vi "Scpi_srend_reply_test.vi"() -> ()   [LabVIEW 2009]
panel:
  out "size(s)":i32
  out "loops":i32
  in  "Commands":string[](array[string])=["*IDN?", ":SYST:VER\u0000S?", ":SERV:SENS:TYPE?"]
  out "Replys":string[](array[string])
  out "error out":errorcluster
  in  "Instrument":T1(ring)
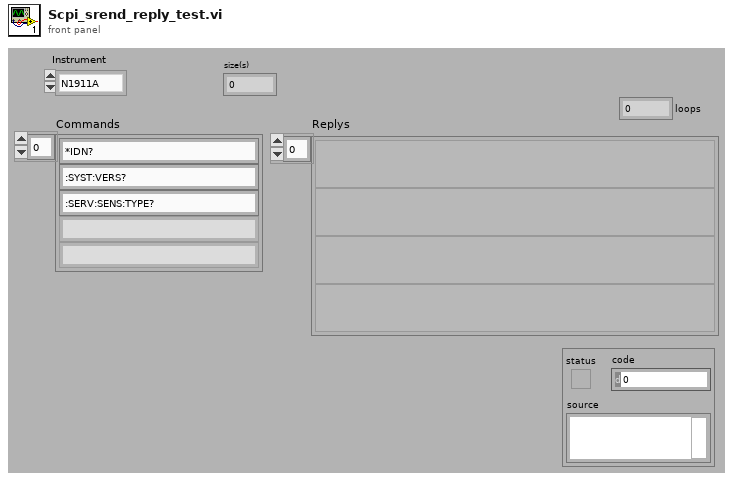
[diagram p1: front panel]
types:
  T1 = enum16{"N1911A", "Siggen", "34980a", "E4418B", "Rvp8"}
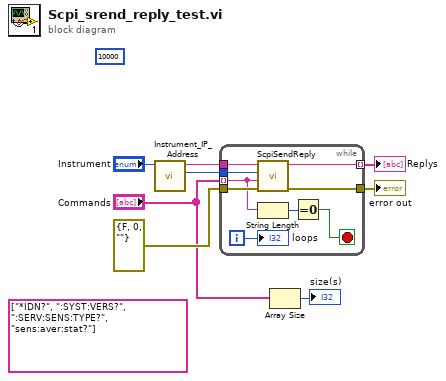
[diagram p0: block diagram]
diagram:
  (unwired) string[] ["*IDN?", ":SYST:VERS?", ":SERV:SENS:TYPE?", "sens:aver:stat?"] ("Commands")
  (unwired) 10000 ("timeout ms (60000)")
  n1 = call "Instrument_IP_Address.vi"("Instrument"="Instrument") -> ("Port"=w6:u16, "IP Address"=w7:string)  [unwired: 9 in]
  n2 = while {
    tunnel: w7 -> [w17]
    tunnel: w6 -> [w16]
    tunnel: "Commands" -> [w12] mode=indexing
    tunnel: errorcluster {"status"=FALSE, "code"=0, "source"=""} ("error in (no error)") -> [w15]
    tunnel: [w14] -> w3 mode=indexing
    tunnel: [w13] -> w4
    i -> [w10]
    stop <- w9 stop-if-true
    n3 = call "ScpiSendReply.vi"("error in (no error)"=w15, "Command"=w12, "TCP port"=w16, "IP Address"=w17) -> ("Error out"=w13:errorcluster, "Reply"=w14:string)  [unwired: 5 in]
    n4 = String Length(string=w12) -> (length=w11:i32)
    n5 = Equal To 0?(x=w11) -> (x = 0?=w9:bool)
    "loops" <- w10
  }
  "error out" <- w4
  "Replys" <- w3
  n6 = Array Size(array="Commands") -> (size(s)=→"size(s)":i32)
